vi "NL_update_2D_Diff_Robot_Pos.vi"(7 "Input Delta s":T1, 9 "Fk":T2 format="%_4e", 11 "state k":T1) -> (1 "Fk+1":T2 format="%_4e", 3 "state k+1":T1)   [LabVIEW 2019]
uses:
  coordinate.ctl
  <vilib>/Analysis/Matrix/Datatypes/RealMatrix.ctl
  <vilib>/Analysis/Matrix/NI_Matrix.lvlib
panel:
  # "x\n\ny\n\ntheta"
  # "Delta s R\n\nDelta s L"
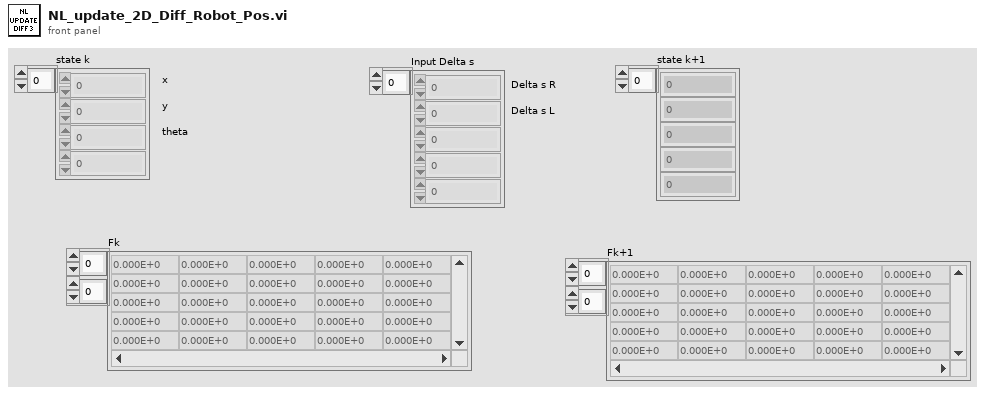
[diagram p1: front panel]
types:
  T1 = typedef "coordinate.ctl" = dbl[]
  T2 = typedef "NI_Matrix.lvlib/RealMatrix.ctl" = dbl[][]
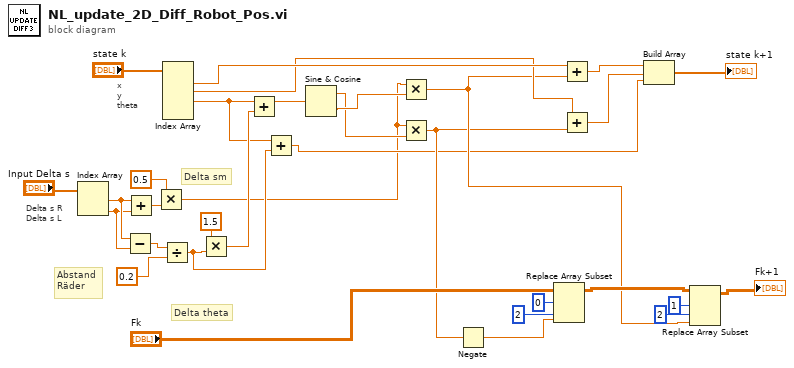
[diagram p0: block diagram]
diagram:
  # "Delta theta"
  # "Delta sm"
  # "Abstand\nRäder"
  # "Delta s R\nDelta s L"
  # "x\ny\ntheta"
  n1 = Index Array(array="Input Delta s") -> (element #1=w13:dbl, element #2=w12:dbl)  [unwired: 2 in]
  n2 = Subtract(x=w13, y=w12) -> (x-y=w11:dbl)
  n3 = Add(x=w13, y=w12) -> (x+y=w9:dbl)
  n4 = Multiply(x=0.5, y=w9) -> (x*y=w1:dbl)
  n5 = Divide(x=w11, y=0.2) -> (x/y=w3:dbl)
  n6 = Index Array(array="state k") -> (element #1=w29:dbl, element #2=w28:dbl, element #3=w4:dbl)  [unwired: 5 in, 2 out]
  n7 = Multiply(x=1.5, y=w3) -> (x*y=w5:dbl)
  n8 = Add(x=w4, y=w5) -> (x+y=w6:dbl)
  n9 = Add(x=w4, y=w3) -> (x+y=w2:dbl)
  n10 = Sine & Cosine(0:w6) -> (1:w30:dbl, 2:w31:dbl)
  n11 = Multiply(x=w1, y=w31) -> (x*y=w16:dbl)
  n12 = Multiply(x=w1, y=w30) -> (x*y=w15:dbl)
  n13 = Negate(x=w15) -> (-x=w21:dbl)
  n14 = Replace Array Subset(array="Fk", new element=w21, index (row)=0, index (col)=2 ("disabled index (col)")) -> (w20:T2)
  n15 = Add(x=w29, y=w16) -> (x+y=w27:dbl)
  n16 = Add(x=w28, y=w15) -> (x+y=w25:dbl)
  n17 = Build Array(w27, w25, w2) -> (→"state k+1":dbl[])
  n18 = Replace Array Subset(array=w20, new element=w16, index (row)=1, index (col)=2 ("disabled index (col)")) -> (→"Fk+1":T2)
